vi "RegisterLicense.vi"(8 "key":string, 9 "Licensee":string, 11 "error in (no error)":errorcluster) -> (0 "License state":string, 1 "State":i32(ring) items=["Invalid"=0, "Trial"=1, "ExtraTrial"=2, "Expired"=3, "MaintenanceNeeded"=4, "Licensed"=5, "None"=-1], 3 "error out":errorcluster)   [LabVIEW 2014, in "UnderAutomation.Yaskawa.lvlib"]
uses:
  UnderAutomation.Yaskawa.lvlib
  C:/Users/fg/Documents/Yaskawa.vi/LabVIEW_2024/UnderAutomation.Yaskawa/lib/UnderAutomation.Yaskawa.dll
  LabVIEW_2024/UnderAutomation.Yaskawa/lib/UnderAutomation.Yaskawa.dll
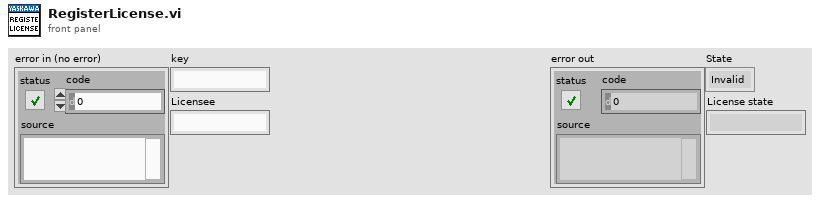
[diagram p1: front panel]
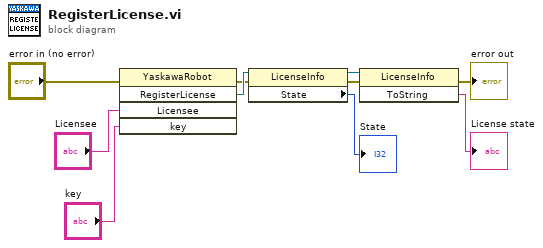
[diagram p0: block diagram]
diagram:
  n1 = invoke class="YaskawaRobot" method="RegisterLicense"(error in="error in (no error)", "Licensee"="Licensee", "key"="key") -> (error out=w8:errorcluster, "RegisterLicense"=w9:refnum<k24>)  [unwired: 2 in, 3 out]
  n2 = property class="LicenseInfo"(reference=w9, error in=w8) -> (reference out=w5:refnum<k24>, error out=w1:errorcluster, "State"=→"State":i32)
  n3 = invoke class="LicenseInfo" method="ToString"(reference=w5, error in=w1) -> (error out=→"error out":errorcluster, "ToString"=→"License state":string)  [unwired: 1 in, 1 out]
